vi "Cache-GEvt Filter Object.vi"() -> (3 "CSM:LogFilter.lvclass":refnum<class "LogFilter.lvclass">)   [LabVIEW 2017, in "Communicable State Machine.lvlib"]
doc: "### Cache-GEvt Filter Object.vi\n\n-- <b>Indicators</b> --\n- <b>CSM:LogFilter.lvclass</b>:"
uses:
  Communicable State Machine.lvlib
  LogFilter/LogFilter.lvclass
  ChangeFlag/ChangeFlag-Read.vi
  LogFilter/SettingVIs/Set Periodic Log Filter.vi
  LogFilter/SettingVIs/Set CSM Broadcast Filter.vi
  LogFilter/SettingVIs/Set CSM StateType Filter.vi
  LogFilter/SettingVIs/Set Global StateType Filter.vi
  LogFilter/SettingVIs/Set CSM State Filter.vi
  LogFilter/SettingVIs/Set CSM LogType Filter.vi
  LogFilter/SettingVIs/Set Global Broadcast Filter.vi
  LogFilter/SettingVIs/Set Global State Filter.vi
  LogFilter/SettingVIs/Set Global LogType Filter.vi
  LogFilter/SettingVIs/Set Global CSM Filter.vi
  ChangeFlag/ChangeFlagDB.vi
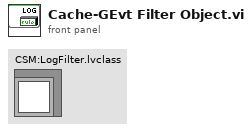
[diagram p1: front panel]
types:
  T1 = typedef "Communicable State Machine.lvlib/_CSM_GlobalLog Filter Rules - v1.2.ctl" = cluster{"Global":cluster{"CSM":string[], "LogType":T2[], "State":string[], "StateType":T3[], "Broadcast":string[]}, "CSM":cluster{"LogType":cluster{"CSM":string, "LogType":T2}[], "State":cluster{"CSM":string, "State":string}[], "StateType":cluster{"CSM":string, "LogType":T3}[], "Broadcast":cluster{"CSM":string, "Broadcast":string}[]}, "PeriodicMessageFilter":cluster{"Enable":bool, "Threshold(#/s)":dbl, "CheckPeriod(s)":dbl}}
  T2 = typedef "Communicable State Machine.lvlib/_CSM_GlobalLog_MSG_TYPE.ctl" = enum16{"User Log", "State Change", "Status", "Interrupt", "Register", "Unregister", "Error Log", "Module Created", "Module Destroyed", "Async Message", "No-Rep Async Message", "Sync Message", "AsyncMsg Complete", "SyncMsg Complete"}
  T3 = typedef "Communicable State Machine.lvlib/_CSM_GlobalLog_STATE_TYPE.ctl" = enum16{"State - Internal State", "State - External Message", "State - Response", "State - Complete"}
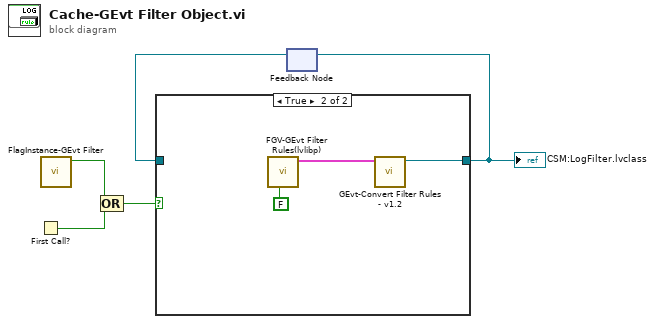
[diagram p0: block diagram]
diagram:
  n1 = First Call?() -> (First Call?: T/F=w5:bool)
  n2 = call "FlagInstance-GEvt Filter.vi"() -> ("Changed"=w1:bool)  [unwired: 10 in, 1 out]
  n3 = Compound Arithmetic op=OR(w1, w5) -> (w4:bool)
  n4 = feedback #1() -> (w2:refnum<class "LogFilter.lvclass">)  [unwired: 1 in]
  n5 = case shown="True" w4 {
    tunnel: [w6 w7] -> w3
    tunnel: w2 -> [w6 _]
    frame False {
    }
    frame True {
      n6 = call "FGV-GEvt Filter Rules(lvlibp).vi"("Set? (T)/Get(F)"=FALSE ("Set(T)/Get(F)")) -> ("Rules-v1.2 out"=w8:T1)  [unwired: 9 in, 1 out]
      n7 = call "GEvt-Convert Filter Rules - v1.2.vi"("Rules-v1.2"=w8) -> ("GlobalLogFilter"=w7:refnum<class "LogFilter.lvclass">)  [unwired: 10 in]
    }
  }
  "CSM:LogFilter.lvclass" <- w3
  n8 = feedback-in #1(w3) -> ()
